vi "Custom Packet Multiple.vi"() -> ()   [LabVIEW 2021]
uses:
  <userlib>/SciSDK/SciSDK_Labview.lvlib
panel:
  out "Counter 3":u32
  out "Counter 2":u32
  out "Counter 1":u32
  out "Counter 0":u32
  out "Timestamp":u32
  out "Header":string
  out "CP Buffer Out":T1
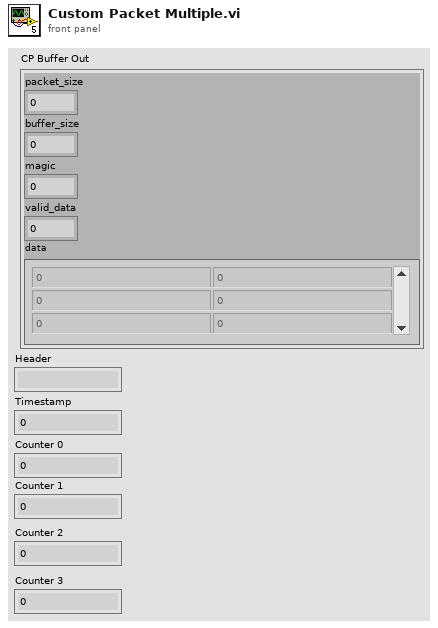
[diagram p1: front panel]
types:
  T1 = cluster{"packet_size":u32, "buffer_size":u32, "magic":u32, "valid_data":dbl, "data":u32[][]}
  T2 = cluster{"Name":string, "Board Model":string, "Handle":u64}
  T3 = cluster{"Board Name":string, "Board Model":string, "SciSDK Handle":u64}
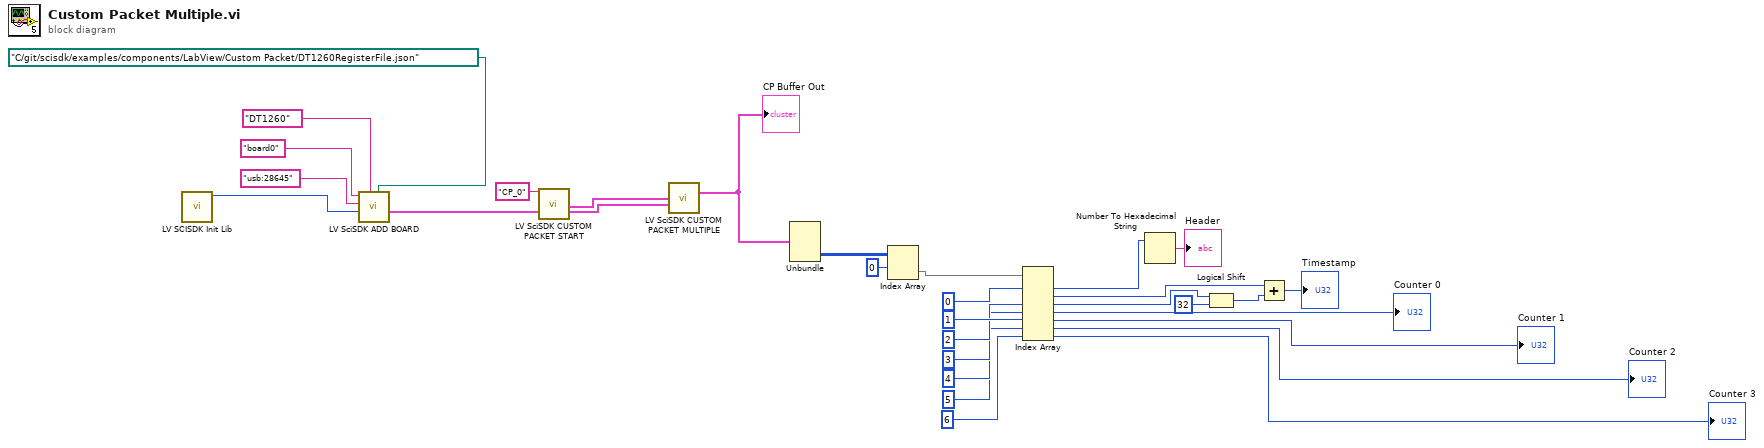
[diagram p0: block diagram]
diagram:
  n1 = call <userlib>:"LV SCISDK Init Lib.vi"() -> ("function return"=w31:u64)  [unwired: 11 in]
  n2 = call <userlib>:"LV SciSDK ADD BOARD.vi"("JsonFile"=path "C:/git/scisdk/examples/components/LabView/Custom Packet/DT1260RegisterFile.json", "Board Model"="DT1260", "SciSDK Handle"=w31, "DevicePath"="usb:28645", "Name"="board0") -> ("Board Handle Out"=w26:T2)  [unwired: 4 in, 2 out]
  n3 = call <userlib>:"LV SciSDK CUSTOM PACKET START.vi"("Custom Packet Name"="CP_0", "Handle In"=w26) -> ("CP Handle Out"=w23:cluster{"CP Path":string, "CP Name":string}, "Board Handle Out"=w24:T3)  [unwired: 15 in, 1 out]
  n4 = call <userlib>:"LV SciSDK CUSTOM PACKET MULTIPLE.vi"("CP Handle In"=w23, "Handle In"=w24) -> ("CP Buffer Out"=w22:T1)  [unwired: 9 in, 4 out]
  "CP Buffer Out" <- w22
  n5 = Unbundle(w22) -> ("data"=w21:u32[][])  [unwired: 4 out]
  n6 = Index Array(array=w21, index (row)=0) -> (element=w19:u32[])  [unwired: 1 in]
  n7 = Index Array(array=w19, index #1=0 ("index"), index #2=1 ("index"), index #3=2 ("index"), index #4=3 ("index"), index #5=4 ("index"), index #6=5 ("index"), index #7=6 ("index")) -> (element #1=w11:u32, element #2=w6:u32, element #3=w8:u32, element #4=→"Counter 0":u32, element #5=→"Counter 1":u32, element #6=→"Counter 2":u32, element #7=→"Counter 3":u32)
  n8 = Number To Hexadecimal String(2:w11) -> (0:→"Header":string)  [unwired: 1 in]
  n9 = Logical Shift(y=w8, x=u32 32) -> (x << y=w7:u32)
  n10 = Add(x=w6, y=w7) -> (x+y=→"Timestamp":u32)
